vi "Draw.vi"(8 "error in (no error)":errorcluster, 9 "disable contained items?":bool, 10 "IB_Tree":refnum<class "IB_Tree.lvclass">, 11 "IB_TreeProjContainer in":refnum<class "IB_Tree_Item_Proj_Container.lvclass">) -> (0 "error out":errorcluster, 3 "IB_TreeProjContainer out":refnum<class "IB_Tree_Item_Proj_Container.lvclass">)   [LabVIEW 2020, in "IB_Tree_Item_Proj_Container.lvclass"]
uses:
  <vilib>/AppBuilder/IB_Classes/Tree_Item_Proj_Container/IB_Tree_Item_Proj_Container.lvclass
  <vilib>/AppBuilder/IB_Classes/Tree_Item_Proj_Container/IB_Tree_Item_Proj_Container.lvclass/IB_Tree_Item_Proj_Container.ctl
  <vilib>/AppBuilder/IB_Classes/Tree_Item_Proj/IB_Tree_Item_Proj.lvclass
  <vilib>/AppBuilder/IB_Classes/Tree/IB_Tree.lvclass
  <vilib>/AppBuilder/IB_Classes/Tree_Item/IB_Tree_Item.lvclass
  e:/builds/penguin/labview/branches/2020/dev/dist/vi.lib/AppBuilder/IB_Classes/Tree_Item_Proj/IB_Tree_Item_Proj.lvclass
  e:/builds/penguin/labview/branches/2020/dev/dist/vi.lib/AppBuilder/IB_Classes/Tree_Item/IB_Tree_Item.lvclass
  e:/builds/penguin/labview/branches/2020/dev/dist/vi.lib/AppBuilder/IB_Classes/Tree_Item_Proj_Container/IB_Tree_Item_Proj_Container.lvclass
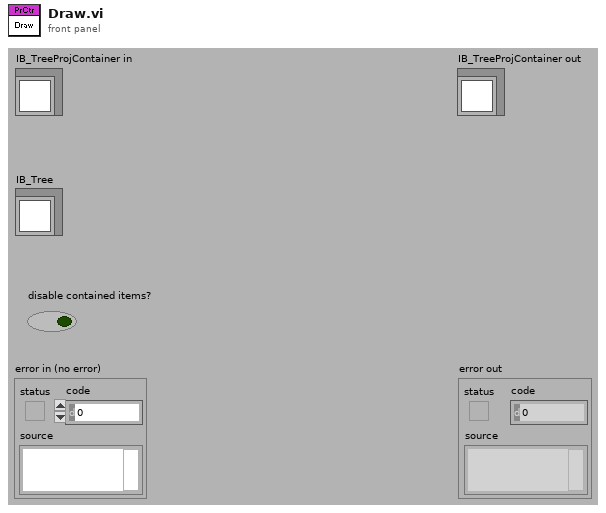
[diagram p1: front panel]
types:
  T1 = typedef "IB_Tree_Item.ctl" = cluster{"symbol index":i32, "child tag":string, "parentTag":string, "left cell name":string}
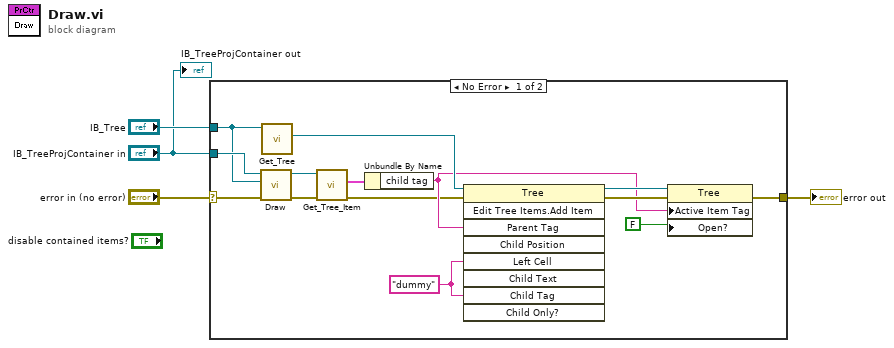
[diagram p0: block diagram]
diagram:
  n1 = case shown="No Error" "error in (no error)" {
    selector: "error in (no error)" -> [w15 w19]
    tunnel: [w11 w19] -> w3
    tunnel: "IB_Tree" -> [w10 _]
    tunnel: "IB_TreeProjContainer in" -> [w18 _]
    frame No Error {
      w17 = "dummy" ("Left Cell String")
      n2 = call-parent "Draw.vi"("error in (no error)"=w15, "IB_Tree"=w10, "IB_TreeItem in"=w18) -> ("error out"=w6:errorcluster, "IB_TreeItem out"=w8:refnum<class "IB_Tree_Item_Proj_Container.lvclass">)  [unwired: 1 in, 6 out]
      n3 = call <vilib>:"Get_Tree.vi"("IB_Tree in"=w10) -> ("ctl"=w14:refnum<vi>)  [unwired: 1 in, 9 out]
      n4 = call <vilib>:"Get_Tree_Item.vi"("error in (no error)"=w6, "IB_TreeItem in"=w8) -> ("error out"=w5:errorcluster, "data"=w9:T1)  [unwired: 8 out]
      n5 = Unbundle By Name(w9) -> ("child tag"=w7:string)
      n6 = invoke class="Tree" method="Edit Tree Items.Add Item"(reference=w14, error in=w5, "Parent Tag"=w7, "Left Cell"=w17, "Child Tag"=w17) -> (reference out=w13:refnum<vi>, error out=w12:errorcluster)  [unwired: 4 in, 7 out]
      n7 = property class="Tree"(reference=w13, error in=w12, "Active Item Tag"=w7, "Open?"=FALSE ("Active Item:Open?")) -> (error out=w11:errorcluster)  [unwired: 1 out]
    }
    frame Error {
    }
  }
  "error out" <- w3
  "IB_TreeProjContainer out" <- "IB_TreeProjContainer in"
